vi "Check Parameters.vi"(8 "error in (no error)":errorcluster, 11 "link in":refnum<class "NI_Robotics_Link.lvclass">) -> (0 "error out":errorcluster, 1 "dynamics valid":bool, 2 "kinematics valid":bool, 3 "lin out":refnum<class "NI_Robotics_Link.lvclass">)   [LabVIEW 2017, in "NI_Robotics_Link.lvclass"]
uses:
  <vilib>/robotics/Kinematics/Link/NI_Robotics_Link.lvclass
  <vilib>/robotics/Kinematics/Link/NI_Robotics_Link.lvclass/NI_Robotics_Link.ctl
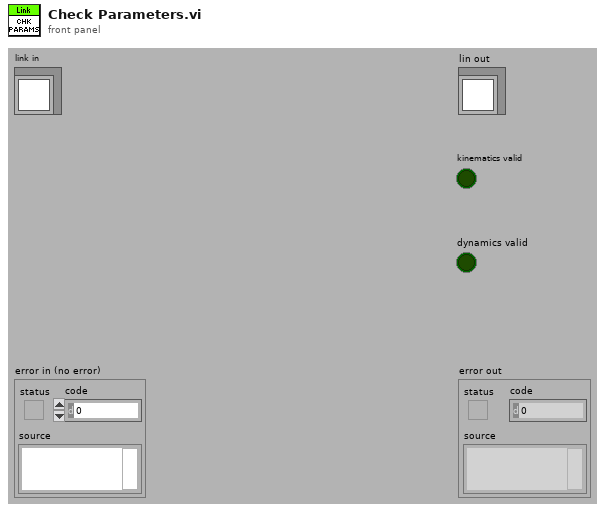
[diagram p1: front panel]
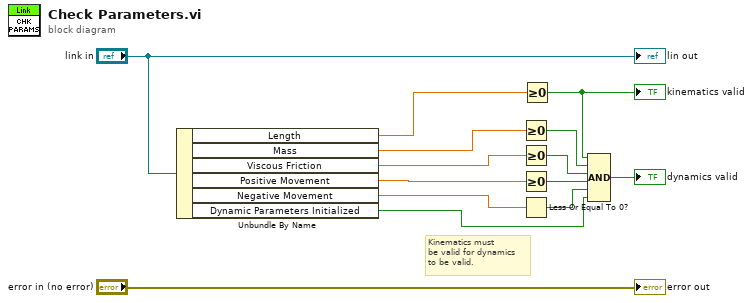
[diagram p0: block diagram]
diagram:
  # "Kinematics must\nbe valid for dynamics\nto be valid."
  n1 = Unbundle By Name("link in") -> ("Length"=w11:dbl, "Mass"=w10:dbl, "Viscous Friction"=w9:dbl, "Positive Movement"=w8:dbl, "Negative Movement"=w7:dbl, "Dynamic Parameters Initialized"=w2:bool)
  n2 = Greater Or Equal To 0?(x=w10) -> (x >= 0?=w6:bool)
  n3 = Greater Or Equal To 0?(x=w9) -> (x >= 0?=w5:bool)
  n4 = Greater Or Equal To 0?(x=w8) -> (x >= 0?=w3:bool)
  n5 = Less Or Equal To 0?(x=w7) -> (x <= 0?=w4:bool)
  n6 = Greater Or Equal To 0?(x=w11) -> (x >= 0?=w1:bool)
  "kinematics valid" <- w1
  n7 = Compound Arithmetic op=AND(w1, w6, w5, w3, w4, w2) -> (→"dynamics valid":bool)
  "error out" <- "error in (no error)"
  "lin out" <- "link in"
